vi "Add KeyValue Pair.vi"(8 "error in (no error)":errorcluster, 9 "value":variant, 10 "key":string, 11 "Leaf in":refnum<class "Leaf.lvclass">) -> (0 "error out":errorcluster, 3 "Leaf out":refnum<class "Leaf.lvclass">)   [LabVIEW 2021, in "Bananas.lvlib" / "Leaf.lvclass"]
uses:
  Leaf.lvclass
  <vilib>/LabVIEW Open Source Project/Data Manipulation/Variant/OpenVariant.lvlib
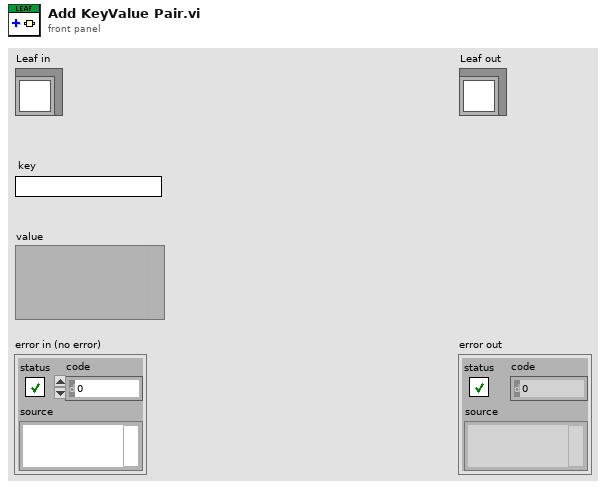
[diagram p1: front panel]
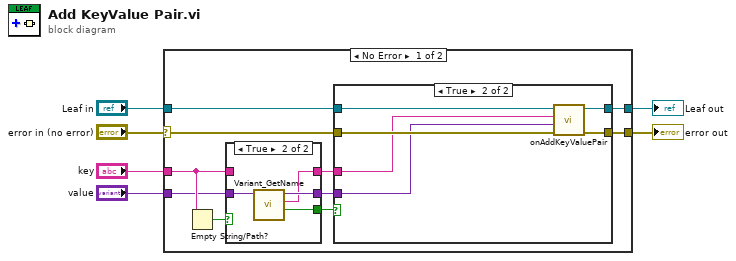
[diagram p0: block diagram]
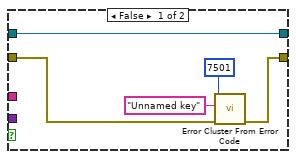
[diagram p2: hidden frame]
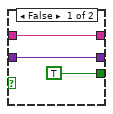
[diagram p3: hidden frame]
diagram:
  n1 = case shown="No Error" "error in (no error)" {
    selector: "error in (no error)" -> [w15 w36]
    tunnel: [w13 w36] -> w5
    tunnel: [w14 w35] -> w3
    tunnel: "Leaf in" -> [w16 w35]
    tunnel: "key" -> [w11 _]
    tunnel: "value" -> [w8 _]
    frame No Error {
      n2 = Empty String/Path?(string/path=w11) -> (empty?=w12:bool)
      n3 = case shown="True" w12 {
        tunnel: w11 -> [w30 _]
        tunnel: [w30 w32] -> w10
        tunnel: [w29 w33] -> w9
        tunnel: w8 -> [w29 w34]
        tunnel: [TRUE ("found") w31] -> w7
        frame False {
        }
        frame True {
          n4 = call <vilib>:"Variant_GetName.vi"("Variant"=w34) -> ("found"=w31:bool, "Name"=w32:string, "Variant dup"=w33:variant)  [unwired: 8 in]
        }
      }
      n5 = case shown="True" w7 {
        tunnel: w16 -> [w21 w27]
        tunnel: w15 -> [w19 w26]
        tunnel: [w21 w25] -> w14
        tunnel: [w20 w24] -> w13
        tunnel: w10 -> [_ w23]
        tunnel: w9 -> [_ w22]
        frame False {
          n6 = call <vilib>:"Error Cluster From Error Code.vi"("error in (no error)"=w19, "error message (\"\")"="Unnamed key" ("error message (\"\")"), "error code (0)"=7501) -> ("error out"=w20:errorcluster)  [unwired: 6 in]
        }
        frame True {
          n7 = call-dynamic "onAddKeyValuePair.vi"("error in (no error)"=w26, "value"=w22, "key"=w23, "Leaf in"=w27) -> ("error out"=w24:errorcluster, "Leaf out"=w25:refnum<class "Leaf.lvclass">)  [unwired: 6 in]
        }
      }
    }
    frame Error {
    }
  }
  "error out" <- w5
  "Leaf out" <- w3
